vi "Celsius To Far.vi"(10 "TempC":dbl) -> (2 "TempF":dbl)   [LabVIEW 2020]
doc: "TempC is input. It takes input temperature in Celsius and It wll provide output in Far"
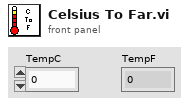
[diagram p1: front panel]
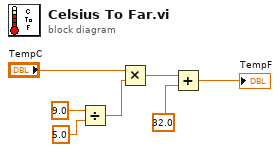
[diagram p0: block diagram]
diagram:
  n1 = Divide(x=9.0, y=5.0 ("x")) -> (x/y=w2:dbl)
  n2 = Multiply(x="TempC", y=w2) -> (x*y=w5:dbl)
  n3 = Add(x=w5, y=32.0 ("x")) -> (x+y=→"TempF":dbl)
